vi "InsertItem.vi"(8 "Error":errorcluster, 9 "NewElement":T1, 10 "SelectedTag":string, 11 "Tree in":refnum<class "Tree.lvclass">) -> (0 "Error":errorcluster, 1 "StepForward":T2(ring), 2 "StepBack":T2(ring), 3 "Tree out":refnum<class "Tree.lvclass">, 4 "Tag":string)   [LabVIEW 2021, in "Tree.lvlib" / "Tree.lvclass"]
uses:
  Tree.lvclass
  Private/TreeControllerTag.ctl
  Tree.lvclass/Tree.ctl
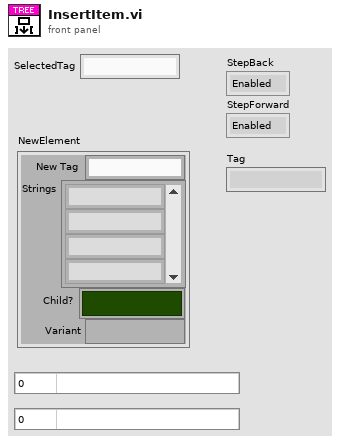
[diagram p1: front panel]
types:
  T1 = cluster{"New Tag":string, "Strings":string[], "Child?":bool, "Variant":variant}
  T2 = enum8{"Enabled", "Disabled", "Disabled and Grayed Out"}
  T3 = cluster{"SelectedTag":string, "New Tag":string, "Strings":string[], "Child?":bool, "Variant":variant}
  T4 = typedef "Tree.lvlib/Tree.lvclass/TreeControllerTag.ctl" = enum8{"Null", "1. Add item", "2. Delete item", "3. Get All Tree Data", "4. Drag Starting", "5. Drag Ended", "6. Add Tree Values", "7. Get Item Value", "8. Edit Item", "9. StepBack", "10. Filter"}
  T5 = cluster{"StepBack":enum8{"Enabled", "Disabled", "Disabled and Grayed Out"}, "StepForward":enum8{"Enabled", "Disabled", "Disabled and Grayed Out"}, "Edit Tree Items:Add Item":string}
  T6 = cluster{"NewElement":cluster{"SelectedTag":string, "New Tag":string, "Strings":string[], "Child?":bool, "Variant":variant}, "queue out":refnum<queue>}
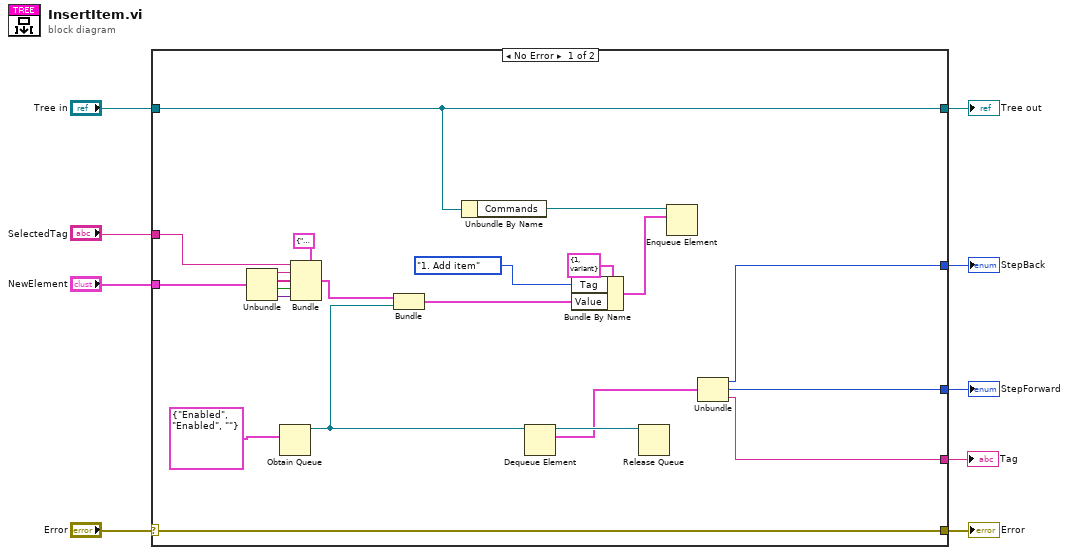
[diagram p0: block diagram]
diagram:
  n1 = case shown="No Error" "Error" {
    selector: "Error" -> [w31 w33]
    tunnel: [w31 w33] -> w8
    tunnel: [w30 w32] -> w6
    tunnel: "Tree in" -> [w30 w32]
    tunnel: [w24 _] -> w5
    tunnel: [w23 _] -> w4
    tunnel: "NewElement" -> [w14 _]
    tunnel: [w21 _] -> w2
    tunnel: "SelectedTag" -> [w15 _]
    frame No Error {
      n2 = Unbundle(w14) -> ("New Tag"=w13:string, "Strings"=w12:string[], "Child?"=w11:bool, "Variant"=w10:variant)
      n3 = Obtain Queue(element data type=T5 {"StepBack"=enum."Enabled", "StepForward"=enum."Enabled", "Edit Tree Items:Add Item"=""} ("output cluster")) -> (queue out=w27:refnum<queue>)  [unwired: 4 in, 2 out]
      n4 = Bundle(cluster=T3 {"SelectedTag"="", "New Tag"="", "Strings"=[], "Child?"=FALSE, "Variant"=variant} ("NewElement"), "SelectedTag"=w15, "New Tag"=w13, "Strings"=w12, "Child?"=w11, "Variant"=w10) -> (w16:T3)
      n5 = Bundle("NewElement"=w16, "queue out"=w27) -> (w28:T6)  [unwired: 1 in]
      n6 = Unbundle By Name(w30) -> ("Commands"=w29:refnum<queue>)
      n7 = Dequeue Element(queue=w27) -> (queue out=w26:refnum<queue>, element=w25:T5)  [unwired: 2 in, 2 out]
      n8 = Bundle By Name(cluster=cluster{"Tag":u8, "Value":variant} {"Tag"=1, "Value"=variant} ("element"), "Tag"=TreeControllerTag."1. Add item", "Value"=w28) -> (w19:cluster{"Tag":u8, "Value":variant})
      n9 = Release Queue(queue=w26) -> ()  [unwired: 2 in, 3 out]
      n10 = Enqueue Element(queue=w29, element=w19) -> ()  [unwired: 2 in, 3 out]
      n11 = Unbundle(w25) -> ("StepBack"=w23:T2, "StepForward"=w24:T2, "Edit Tree Items:Add Item"=w21:string)
    }
    frame Error {
    }
  }
  "Error" <- w8
  "Tree out" <- w6
  "StepForward" <- w5
  "StepBack" <- w4
  "Tag" <- w2
